vi "Download_Config.vi"(8 "error in":errorcluster, 11 "VISA in":refnum<visa-resource-name>) -> (0 "error out":errorcluster, 3 "VISA Refnum out":refnum<visa-resource-name>)   [LabVIEW 2019]
uses:
  SiPM_Tests_Global_Var.vi
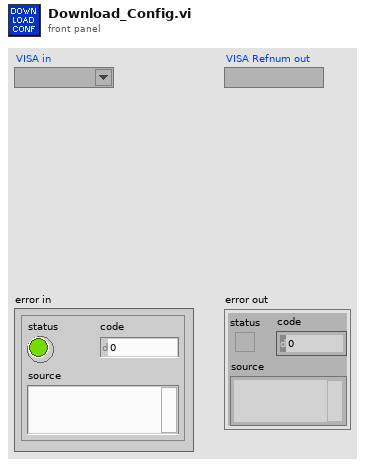
[diagram p1: front panel]
types:
  T1 = enum16{"Channel 1", "Channel 2", "Channel 3", "Channel 4", "Channel 5", "Channel 6"}
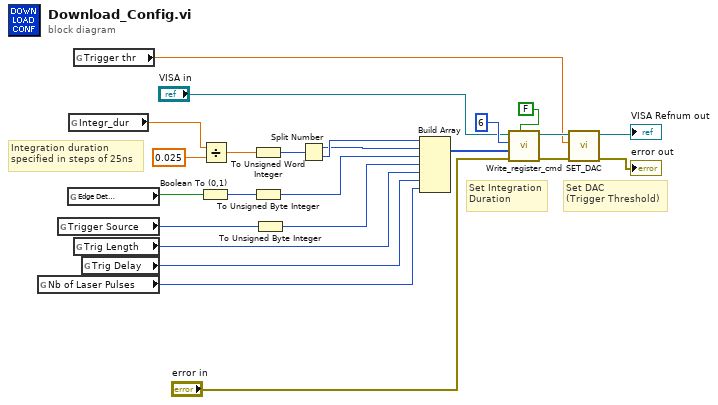
[diagram p0: block diagram]
diagram:
  # "Set DAC \n(Trigger Threshold)"
  # "Set Integration\nDuration"
  # "Integration duration\nspecified in steps of 25ns"
  n1 = global read "SiPM_Tests_Global_Var.vi" "Nb of Laser Pulses"() -> (w3:u8)
  n2 = global read "SiPM_Tests_Global_Var.vi" "Trigger Source"() -> (w2:T1)
  n3 = global read "SiPM_Tests_Global_Var.vi" "Edge Det\nDis"() -> (w9:bool)
  n4 = global read "SiPM_Tests_Global_Var.vi" "Integr_dur"() -> (w10:sgl)
  n5 = global read "SiPM_Tests_Global_Var.vi" "Trigger thr"() -> (w11:sgl)
  n6 = global read "SiPM_Tests_Global_Var.vi" "Trig Length"() -> (w5:u8)
  n7 = global read "SiPM_Tests_Global_Var.vi" "Trig Delay"() -> (w4:u8)
  n8 = Boolean To (0,1)(Boolean=w9) -> (0, 1=w13:i16)
  n9 = Divide(x=w10, y=0.025) -> (x/y=w14:dbl)
  n10 = To Unsigned Word Integer(number=w14) -> (unsigned 16bit integer=w8:u16)
  n11 = To Unsigned Byte Integer(number=w13) -> (unsigned 8bit integer=w12:u8)
  n12 = To Unsigned Byte Integer(number=w2) -> (unsigned 8bit integer=w1:u8)
  n13 = Split Number(x=w8) -> (hi(x)=w6:u8, lo(x)=w7:u8)
  n14 = Build Array(w7, w6, w12, w1, w5, w4, w3) -> (w17:u8[])
  n15 = call "Write_register_cmd.vi"("Fifo-mode En"=FALSE, "Arty-7 Error In"="error in", "Data Array"=w17, "WrReg Addr"=u8 6 ("WrReg Address 2"), "Arty-7 VISA In"="VISA in") -> ("Arty-7 Error out"=w23:errorcluster, "Arty-7 VISA out"=w22:refnum<visa-resource-name>)  [unwired: 3 in, 2 out]
  n16 = call "SET_DAC.vi"("error in (no error)"=w23, "DAC value"=w11, "VISA Refnum in"=w22) -> ("error out"=→"error out":errorcluster, "VISA Refnum out"=→"VISA Refnum out":refnum<visa-resource-name>)  [unwired: 7 in]
